vi "sub_prepare_outputfiles.vi"(8 "error in":errorcluster, 10 "Dynamic data in":T1, 11 "Input parameters":T2={"Measurement type"=enum."Debug", "Sensor type"=enum."HPK_8in_271ch", "Identifier"="test.txt", "Open after execution?"=FALSE, "Plot after execution?"=FALSE, "Display channel"=0, "Voltage Delay (s)"=0.5, "Switch Delay (s)"=0.01, "VISA resource name source"="", "VISA resource name DMM"="", "VISA resource name LCR"="", "Compliance  Level (A)"=10.0, "Voltage Limit (V)"=1000.0, "Data storage location"="", "Scan voltages"="", "Use source as DMM?"=FALSE, "LCR signal frequenzy (Hz)"=10.0, "DMM device"=enum."Keithley2001", "Sampling number"=1, "Use env. sensors on"=enum."Sensirion sht1x/7x", "Switchboard Handle"=0, "Use Switchboard"=FALSE, "LCR signal voltage (V)"=10000.0, "Repeat"=1, "Scan voltages IV"="", "Scan voltages CV"="", "Hex pad numbers?"=FALSE, "Set measurement type"=enum."Debug", "Custom pad scan"="", "IV voltage Delay (s)"=0.5, "CV voltage Delay (s)"=0.5, "Needle measurement?"=FALSE, "Comments"="test.txt", "LCR signal frequenzy (kHz)"=10.0, "Compliance  Level (uA)"=10.0, "Open Correction Array"=array2304x3[6912 elements], "Current set voltage"=0.0, "Last set voltage"=0.0, "Current channel"=0, "Last OpenCorrection index"=-1, "Total curr/vltg every x steps"=10, "Current channel iteration"=0, "No CV corrections"=FALSE, "Mapfile"="", "Corrfile"="", "IV voltage file"=path "", "CV voltage file"=path "", "IV Switch Delay (s)"=0.01, "CV Switch Delay (s)"=0.01, "Invert polarity"=FALSE, "Set debug dirs"=FALSE, "Is n on p"=FALSE, "Source interlock?"=TRUE, "Voltage file used?"=FALSE, "Pad mask"="", "Mask pad above (uA)"=1.0, "LCR device"=enum."LCR_E4980", "Source device"=enum."Source_2410", "HexPlot binary path"="", "PadReductionFactor"=1.0, "Temperature degC"="", "Fluence [neq]"="", "Annealing [min]"=""} {"CV Switch Delay (s)" format="%#_13g"; "IV Switch Delay (s)" format="%#_13g"; "Last set voltage" format="%#_13g"; "Current set voltage" format="%#_13g"; "CV voltage Delay (s)" format="%#_13g"; "IV voltage Delay (s)" format="%#_13g"; "Voltage Limit (V)" format="%#_13g"; "Voltage Delay (s)" format="%#_13g"; "Switch Delay (s)" format="%#_13g"}) -> (0 "error out":errorcluster, 2 "Dynamic data out":T1, 3 "Input parameters out":T2={"Measurement type"=enum."Debug", "Sensor type"=enum."HPK_8in_271ch", "Identifier"="test.txt", "Open after execution?"=FALSE, "Plot after execution?"=FALSE, "Display channel"=0, "Voltage Delay (s)"=0.5, "Switch Delay (s)"=0.01, "VISA resource name source"="", "VISA resource name DMM"="", "VISA resource name LCR"="", "Compliance  Level (A)"=10.0, "Voltage Limit (V)"=1000.0, "Data storage location"="", "Scan voltages"="", "Use source as DMM?"=FALSE, "LCR signal frequenzy (Hz)"=10.0, "DMM device"=enum."Keithley2001", "Sampling number"=1, "Use env. sensors on"=enum."Sensirion sht1x/7x", "Switchboard Handle"=0, "Use Switchboard"=FALSE, "LCR signal voltage (V)"=10000.0, "Repeat"=1, "Scan voltages IV"="", "Scan voltages CV"="", "Hex pad numbers?"=FALSE, "Set measurement type"=enum."Debug", "Custom pad scan"="", "IV voltage Delay (s)"=0.5, "CV voltage Delay (s)"=0.5, "Needle measurement?"=FALSE, "Comments"="test.txt", "LCR signal frequenzy (kHz)"=10.0, "Compliance  Level (uA)"=10.0, "Open Correction Array"=array2304x3[6912 elements], "Current set voltage"=0.0, "Last set voltage"=0.0, "Current channel"=0, "Last OpenCorrection index"=-1, "Total curr/vltg every x steps"=10, "Current channel iteration"=0, "No CV corrections"=FALSE, "Mapfile"="", "Corrfile"="", "IV voltage file"=path "", "CV voltage file"=path "", "IV Switch Delay (s)"=0.01, "CV Switch Delay (s)"=0.01, "Invert polarity"=FALSE, "Set debug dirs"=FALSE, "Is n on p"=FALSE, "Source interlock?"=TRUE, "Voltage file used?"=FALSE, "Pad mask"="", "Mask pad above (uA)"=1.0, "LCR device"=enum."LCR_E4980", "Source device"=enum."Source_2410", "HexPlot binary path"="", "PadReductionFactor"=1.0, "Temperature degC"="", "Fluence [neq]"="", "Annealing [min]"=""} {"CV Switch Delay (s)" format="%#_13g"; "IV Switch Delay (s)" format="%#_13g"; "Last set voltage" format="%#_13g"; "Current set voltage" format="%#_13g"; "CV voltage Delay (s)" format="%#_13g"; "IV voltage Delay (s)" format="%#_13g"; "Voltage Limit (V)" format="%#_13g"; "Voltage Delay (s)" format="%#_13g"; "Switch Delay (s)" format="%#_13g"})   [LabVIEW 2020]
doc: "Creates folder for data and sets output paths accordingly."
uses:
  input_params.ctl
  data_dynamic.ctl
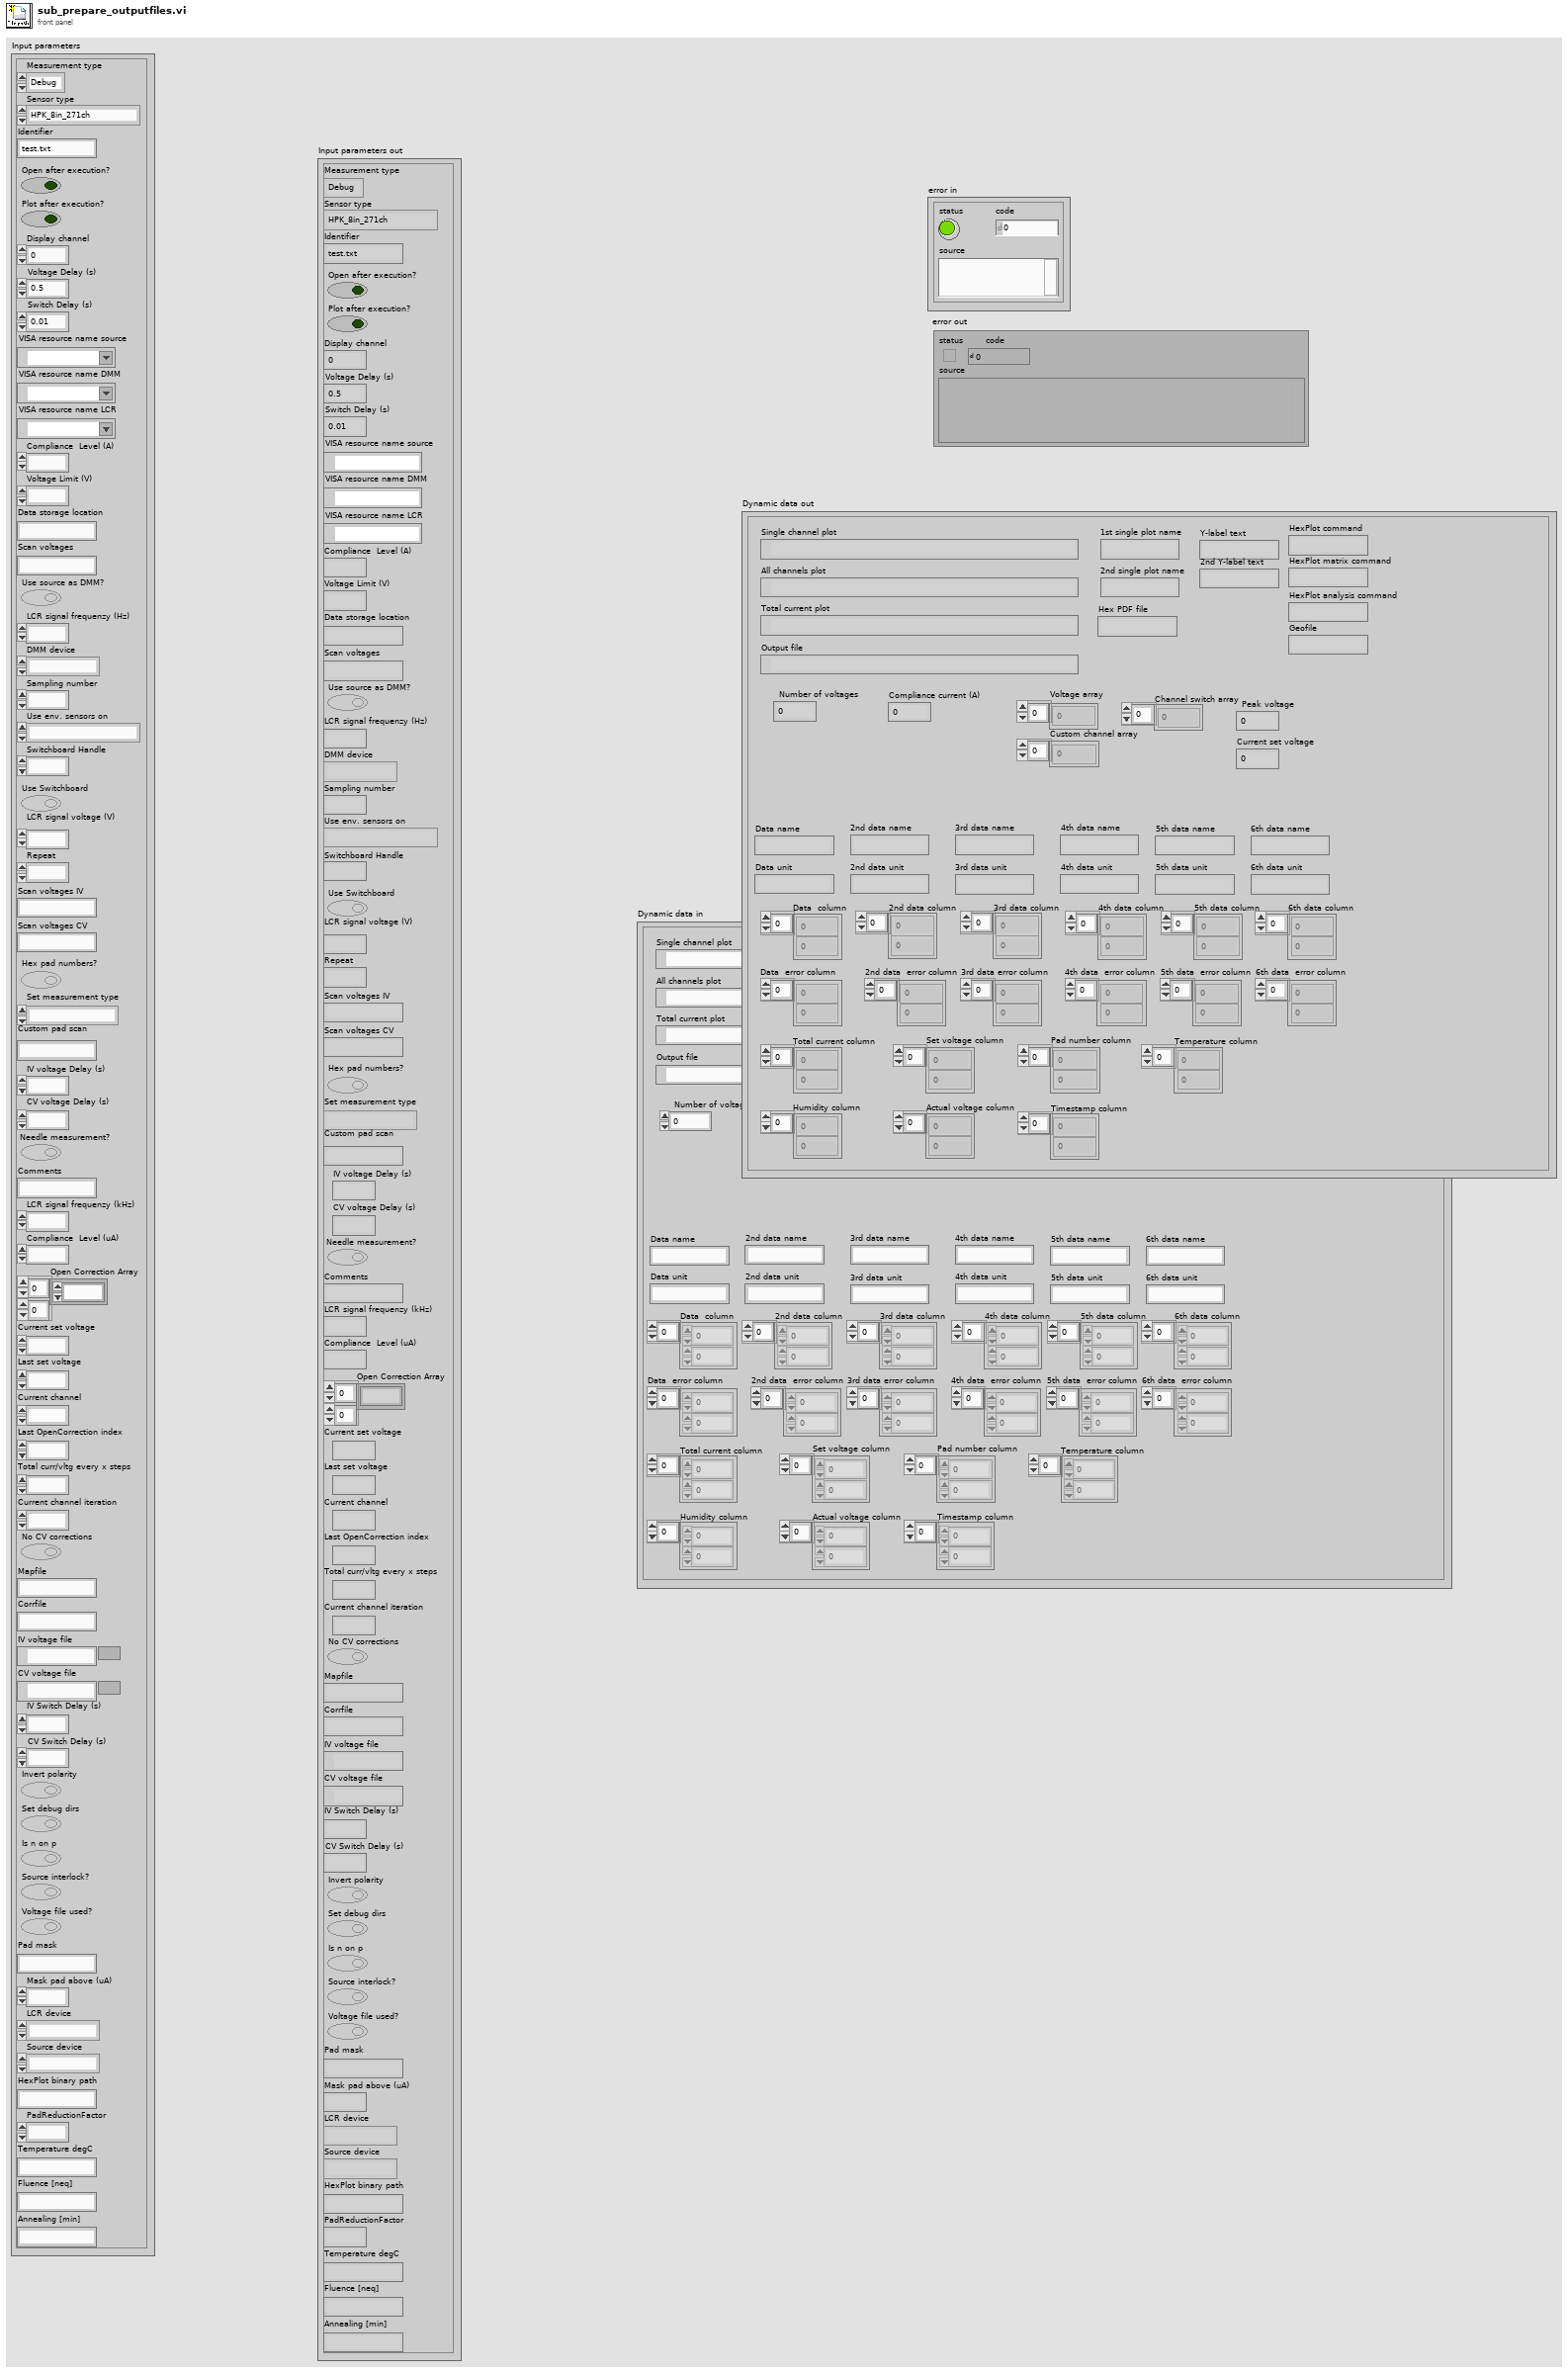
[diagram p1: front panel]
types:
  T1 = typedef "data_dynamic.ctl" = cluster{"Output file":path, "Y-label text":string, "Current set voltage":dbl, "Set voltage column":dbl[], "Pad number column":dbl[], "Data  column":dbl[], "Number of voltages":i32, "Compliance current (A)":dbl, "Geofile":string, "Peak voltage":dbl, "Hex PDF file":string, "Voltage array":dbl[], "Total current column":dbl[], "Timestamp column":dbl[], "Data name":string, "Data unit":string, "2nd data column":dbl[], "2nd data name":string, "2nd data unit":string, "3rd data column":dbl[], "4th data column":dbl[], "3rd data name":string, "3rd data unit":string, "4th data name":string, "4th data unit":string, "Actual voltage column":dbl[], "2nd Y-label text":string, "Single channel plot":path, "Temperature column":dbl[], "Humidity column":dbl[], "Channel switch array":i32[], "1st single plot name":string, "2nd single plot name":string, "All channels plot":path, "HexPlot command":string, "Custom channel array":i32[], "Data  error column":dbl[], "2nd data  error column":dbl[], "3rd data error column":dbl[], "4th data  error column":dbl[], "Total current plot":path, "5th data column":dbl[], "5th data  error column":dbl[], "6th data column":dbl[], "6th data  error column":dbl[], "5th data name":string, "5th data unit":string, "6th data name":string, "6th data unit":string, "HexPlot matrix command":string, "HexPlot analysis command":string}
  T2 = typedef "input_params.ctl" = cluster{"Measurement type":enum16{"IV", "CV", "Debug", "Test_contact"}, "Sensor type":enum16{"HPK_6in_135ch", "HPK_8in_271ch", "IFX_8in_256ch", "Diode", "HPK_6in_239ch", "Full_Matrix", "HPK_8in_271ch_full", "LumiCal", "HPK_8in_444ch", "HPK_8in_198ch_2019", "HPK_8in_MGW_LD_full", "HPK_8in_MGW_LD_a_type_top", "HPK_8in_MGW_LD_a_type_bottom", "HPK_8in_MGW_LD_b_type_left", "HPK_8in_MGW_LD_b_type_right", "HPK_8in_MGW_LD_c_type_left", "HPK_8in_MGW_LD_c_type_right", "HPK_8in_MGW_HD_full", "HPK_8in_MGW_HD_a_type_top", "HPK_8in_MGW_HD_a_type_bottom", "HPK_8in_MGW_HD_b_type_left", "HPK_8in_MGW_HD_b_type_right", "HPK_8in_MGW_HD_c_type_left", "HPK_8in_MGW_HD_c_type_right", "CALICE_6in_256ch"}, "Identifier":string, "Open after execution?":bool, "Plot after execution?":bool, "Display channel":i32, "Voltage Delay (s)":dbl, "Switch Delay (s)":dbl, "VISA resource name source":refnum<visa-resource-name>, "VISA resource name DMM":refnum<visa-resource-name>, "VISA resource name LCR":refnum<visa-resource-name>, "Compliance  Level (A)":dbl, "Voltage Limit (V)":dbl, "Data storage location":string, "Scan voltages":string, "Use source as DMM?":bool, "LCR signal frequenzy (Hz)":dbl, "DMM device":enum16{"Keithley2001", "Keithley2450", "Keithley2410", "Keithley6485", "Keithley6487", "Keithley6517"}, "Sampling number":i32, "Use env. sensors on":enum16{"Sensirion sht1x/7x", "Switch Matrix", "Probecard"}, "Switchboard Handle":u32, "Use Switchboard":bool, "LCR signal voltage (V)":dbl, "Repeat":i32, "Scan voltages IV":string, "Scan voltages CV":string, "Hex pad numbers?":bool, "Set measurement type":enum16{"IV", "CV", "Debug", "Test_contact", "IV+CV"}, "Custom pad scan":string, "IV voltage Delay (s)":dbl, "CV voltage Delay (s)":dbl, "Needle measurement?":bool, "Comments":string, "LCR signal frequenzy (kHz)":dbl, "Compliance  Level (uA)":dbl, "Open Correction Array":dbl[][], "Current set voltage":dbl, "Last set voltage":dbl, "Current channel":i32, "Last OpenCorrection index":i32, "Total curr/vltg every x steps":i32, "Current channel iteration":i32, "No CV corrections":bool, "Mapfile":string, "Corrfile":string, "IV voltage file":path, "CV voltage file":path, "IV Switch Delay (s)":dbl, "CV Switch Delay (s)":dbl, "Invert polarity":bool, "Set debug dirs":bool, "Is n on p":bool, "Source interlock?":bool, "Voltage file used?":bool, "Pad mask":string, "Mask pad above (uA)":dbl, "LCR device":enum16{"LCR_E4980", "AGILENT_4263X"}, "Source device":enum16{"Source_2410", "Source_6487", "Source_2470"}, "HexPlot binary path":string, "PadReductionFactor":dbl, "Temperature degC":string, "Fluence [neq]":string, "Annealing [min]":string}
  T3 = enum16{"HPK_6in_135ch", "HPK_8in_271ch", "IFX_8in_256ch", "Diode", "HPK_6in_239ch", "Full_Matrix", "HPK_8in_271ch_full", "LumiCal", "HPK_8in_444ch", "HPK_8in_198ch_2019", "HPK_8in_MGW_LD_full", "HPK_8in_MGW_LD_a_type_top", "HPK_8in_MGW_LD_a_type_bottom", "HPK_8in_MGW_LD_b_type_left", "HPK_8in_MGW_LD_b_type_right", "HPK_8in_MGW_LD_c_type_left", "HPK_8in_MGW_LD_c_type_right", "HPK_8in_MGW_HD_full", "HPK_8in_MGW_HD_a_type_top", "HPK_8in_MGW_HD_a_type_bottom", "HPK_8in_MGW_HD_b_type_left", "HPK_8in_MGW_HD_b_type_right", "HPK_8in_MGW_HD_c_type_left", "HPK_8in_MGW_HD_c_type_right", "CALICE_6in_256ch"}
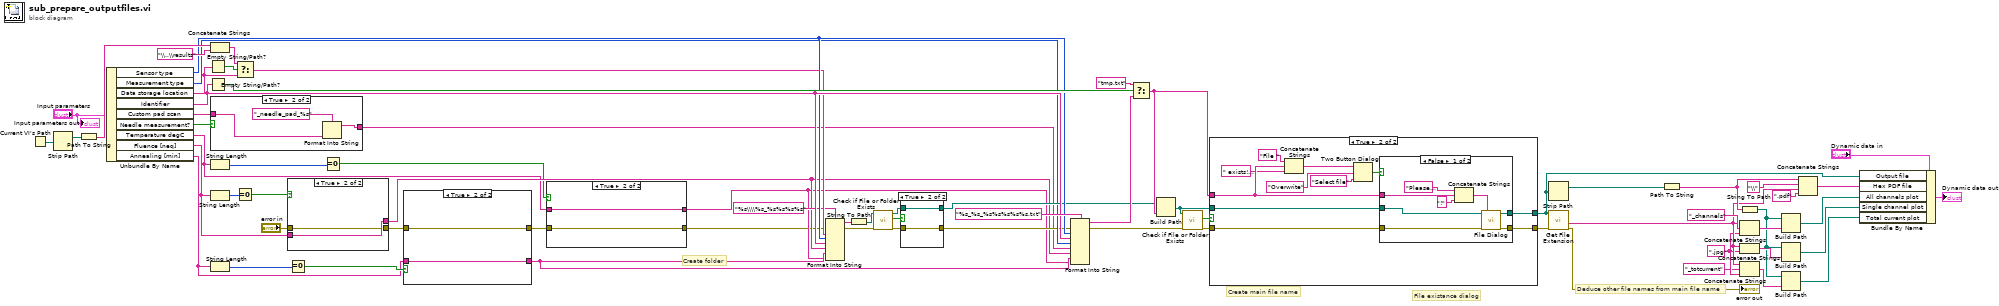
[diagram p0: block diagram]
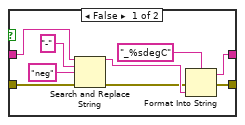
[diagram p2: hidden frame]
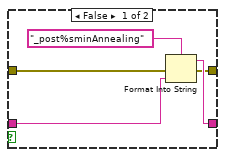
[diagram p3: hidden frame]
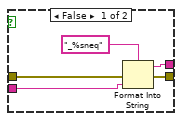
[diagram p4: hidden frame]
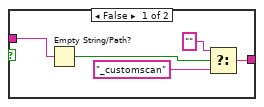
[diagram p5: hidden frame]
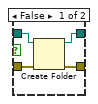
[diagram p6: hidden frame]
diagram:
  w22 = ".jpg" ("string")
  # "Deduce other file names from main file name"
  # "File existance dialog"
  # "Create main file name"
  # "Create folder"
  n1 = Current VI's Path() -> (path=w66:path)
  n2 = Strip Path(path=w66) -> (stripped path=w65:path)  [unwired: 1 out]
  n3 = Path To String(path=w65) -> (string=w64:string)
  n4 = Unbundle By Name("Input parameters") -> ("Sensor type"=w43:T3, "Measurement type"=w35:enum16{"IV", "CV", "Debug", "Test_contact"}, "Data storage location"=w29:string, "Identifier"=w44:string, "Custom pad scan"=w27:string, "Needle measurement?"=w19:bool, "Temperature degC"=w1:string, "Fluence [neq]"=w3:string, "Annealing [min]"=w2:string)
  n5 = Empty String/Path?(string/path=w29) -> (empty?=w67:bool)
  n6 = Empty String/Path?(string/path=w44) -> (empty?=w61:bool)
  n7 = Concatenate Strings(w64, "\\..\\results" ("string")) -> (w62:string)
  n8 = case shown="True" w19 {
    tunnel: w27 -> [w75 w78]
    tunnel: [w71 w77] -> w26
    frame False {
      n9 = Empty String/Path?(string/path=w75) -> (empty?=w74:bool)
      n10 = Select(t="" ("format string"), s=w74, f="_customscan" ("format string")) -> (s? t:f=w71:string)
    }
    frame True {
      n11 = Format Into String(format string="_needle_pad_%s", w78) -> (resulting string=w77:string)  [unwired: 2 in, 1 out]
    }
  }
  n12 = String Length(string=w1) -> (length=w10:i32)
  n13 = String Length(string=w3) -> (length=w17:i32)
  n14 = String Length(string=w2) -> (length=w13:i32)
  n15 = Equal To 0?(x=w17) -> (x = 0?=w16:bool)
  n16 = Select(t=w62, s=w67, f=w29) -> (s? t:f=w42:string)
  n17 = case shown="True" w16 {
    tunnel: w3 -> [w82 w85]
    tunnel: [w81 w85] -> w15
    tunnel: "error in" -> [w80 w84]
    tunnel: [w79 w84] -> w7
    frame False {
      n18 = Format Into String(format string="_%sneq", error in=w80, w82) -> (resulting string=w81:string, error out=w79:errorcluster)  [unwired: 1 in]
    }
    frame True {
    }
  }
  n19 = Equal To 0?(x=w13) -> (x = 0?=w14:bool)
  n20 = Equal To 0?(x=w10) -> (x = 0?=w11:bool)
  n21 = case shown="True" w14 {
    tunnel: w2 -> [w90 w92]
    tunnel: [w88 w92] -> w12
    tunnel: w7 -> [w87 w91]
    tunnel: [w86 w91] -> w6
    frame False {
      n22 = Format Into String(format string="_post%sminAnnealing", error in=w87, w90) -> (resulting string=w88:string, error out=w86:errorcluster)  [unwired: 1 in]
    }
    frame True {
    }
  }
  n23 = case shown="True" w11 {
    tunnel: [w100 w103] -> w9
    tunnel: w1 -> [w97 w103]
    tunnel: w6 -> [w95 w102]
    tunnel: [w93 w102] -> w5
    frame False {
      n24 = Search and Replace String(input string=w97, search string="-", replace string="neg", error in=w95) -> (result string=w96:string, error out=w94:errorcluster)  [unwired: 4 in, 2 out]
      n25 = Format Into String(format string="_%sdegC", error in=w94, w96) -> (resulting string=w100:string, error out=w93:errorcluster)  [unwired: 1 in]
    }
    frame True {
    }
  }
  n26 = Format Into String(format string="%s\\\\%s_%s%s%s%s", error in=w5, w42, w43, w44, w15, w12, w9) -> (resulting string=w41:string, error out=w4:errorcluster)  [unwired: 1 in]
  n27 = String To Path(string=w41) -> (path=w39:path)
  n28 = call <vilib>:"Check if File or Folder Exists.vi"("error in (no error)"=w4, "path"=w39) -> ("error out"=w31:errorcluster, "file or folder exists?"=w38:bool, "dup path"=w37:path)  [unwired: 7 in]
  n29 = case shown="True" w38 {
    tunnel: w37 -> [w107 w109]
    tunnel: [w106 w109] -> w36
    tunnel: w31 -> [w105 w108]
    tunnel: [w104 w108] -> w30
    frame False {
      n30 = Create Folder(path (use dialog)=w107, error in=w105) -> (created path=w106:path, error out=w104:errorcluster)  [unwired: 1 in, 1 out]
    }
    frame True {
    }
  }
  n31 = Format Into String(format string="%s_%s_%s%s%s%s%s.txt", error in=w30, w43, w44, w35, w26, w15, w12, w9) -> (resulting string=w58:string, error out=w45:errorcluster)  [unwired: 1 in]
  n32 = Select(t="tmp.txt", s=w61, f=w58) -> (s? t:f=w55:string)
  n33 = Build Path(base path=w36, name or relative path=w55) -> (appended path=w57:path)
  n34 = call <vilib>:"Check if File or Folder Exists.vi"("error in (no error)"=w45, "path"=w57) -> ("error out"=w56:errorcluster, "file or folder exists?"=w18:bool)  [unwired: 7 in, 1 out]
  n35 = case shown="True" w18 {
    tunnel: w57 -> [w111 w122]
    tunnel: [w111 w121] -> w54
    tunnel: w56 -> [w110 w120]
    tunnel: [w110 w119] -> w50
    tunnel: w55 -> [_ w118]
    frame False {
    }
    frame True {
      n36 = Concatenate Strings("File " ("string"), w118, " exists! Overwite?" ("string")) -> (w115:string)
      n37 = Two Button Dialog(message=w115, 1:"Select file" ("Center Button Text (\"No\")"), 2:"Overwrite" ("Left Button Text (\"Yes\")")) -> (T button?=w112:bool)
      n38 = case shown="False" w112 {
        tunnel: w122 -> [w130 w132]
        tunnel: [w129 w132] -> w121
        tunnel: w120 -> [w128 w131]
        tunnel: [w127 w131] -> w119
        tunnel: w118 -> [w124 _]
        frame False {
          n39 = Concatenate Strings("Please chose a new file instead of  " ("prompt (Choose or enter file path)"), w124, "!" ("string")) -> (w126:string)
          n40 = call "File Dialog"("start path"=w130, "prompt"=w126, "error in"=w128) -> ("selected path"=w129:path, "error out"=w127:errorcluster)  [unwired: 9 in, 2 out]
        }
        frame True {
        }
      }
    }
  }
  n41 = Strip Path(path=w54) -> (stripped path=w69:path)  [unwired: 1 out]
  n42 = call <vilib>:"Get File Extension.vi"("error in (no error)"=w50, "file"=w54) -> ("error out"=→"error out":errorcluster, "filename without extension"=w23:string)  [unwired: 5 in, 3 out]
  n43 = Path To String(path=w69) -> (string=w51:string)
  n44 = String To Path(string=w51) -> (path=w25:path)
  n45 = Concatenate Strings(w23, "_channels" ("string"), w22) -> (w49:string)
  n46 = Concatenate Strings(w23, w22) -> (w52:string)
  n47 = Concatenate Strings(w23, "_totcurrent" ("string"), w22) -> (w24:string)
  n48 = Build Path(base path=w25, name or relative path=w49) -> (appended path=w46:path)
  n49 = Build Path(base path=w25, name or relative path=w52) -> (appended path=w47:path)
  n50 = Build Path(base path=w25, name or relative path=w24) -> (appended path=w20:path)
  n51 = Concatenate Strings(w51, "\\" ("string"), w23, ".pdf" ("string")) -> (w53:string)
  n52 = Bundle By Name(cluster="Dynamic data in", "Output file"=w54, "Hex PDF file"=w53, "All channels plot"=w46, "Single channel plot"=w47, "Total current plot"=w20) -> (→"Dynamic data out":T1)
  "Input parameters out" <- "Input parameters"
